vi "Password Protection.vi"(7 "Action (Validate)":T1=enum."Validate Password", 8 "error in":errorcluster, 11 "configuration file path":path) -> (0 "error out":errorcluster, 3 "Validated?":bool)   [LabVIEW 2018, in "Password Protection.lvlib"]
uses:
  Password Protection.lvlib
  Controls/State Machine.ctl
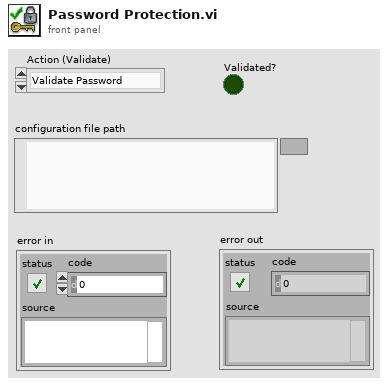
[diagram p1: front panel]
types:
  T1 = typedef "Password Protection.lvlib/State Machine.ctl" = enum16{"Prompt for Password", "Validate Password", "Check Expiration", "Renew Expiration", "Logout", "Stop"}
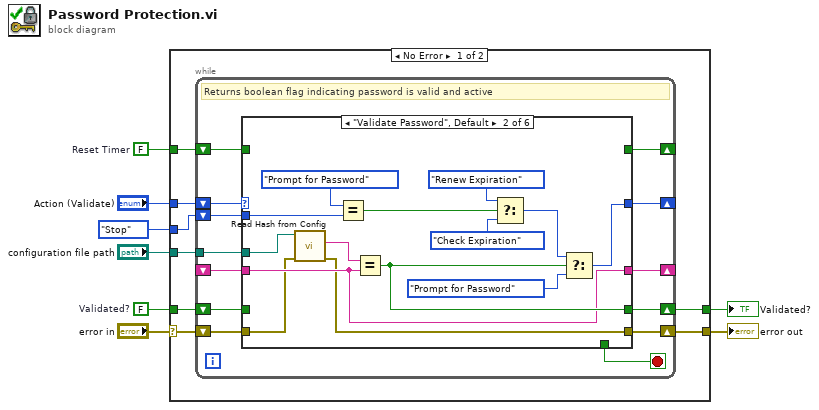
[diagram p0: block diagram]
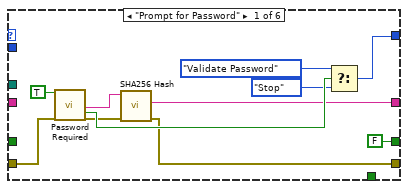
[diagram p2: hidden frame]
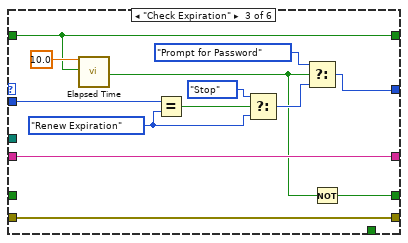
[diagram p3: hidden frame]
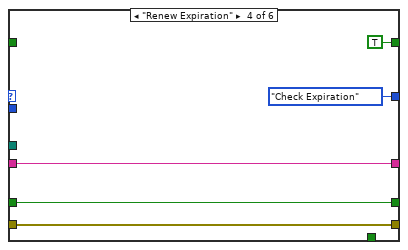
[diagram p4: hidden frame]
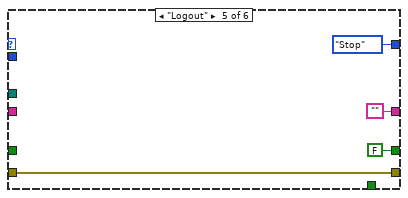
[diagram p5: hidden frame]
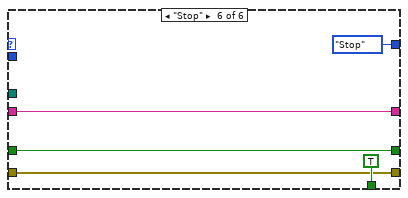
[diagram p6: hidden frame]
diagram:
  w5 = FALSE  # Reset Timer
  w7 = FALSE  # Validated?
  n1 = case shown="No Error" "error in" {
    selector: "error in" -> [w9 w82]
    tunnel: "Action (Validate)" -> [w16 _]
    tunnel: w7 -> [w15 _]
    tunnel: [w14 _] -> w6
    tunnel: w5 -> [w13 _]
    tunnel: State_Machine."Stop" ("f") -> [w12 _]
    tunnel: "configuration file path" -> [w11 _]
    tunnel: [w10 w82] -> w1
    frame No Error {
      n2 = while {
        shift-right: [w28] -> _
        shift-left: _ -> [w29]
        shift-right: [w26] -> _
        shift-left: w16 -> [w27]
        shift-right: [w24] -> w14
        shift-left: w15 -> [w25]
        shift-right: [w22] -> _
        shift-left: w13 -> [w23]
        shift-left: w12 -> [w21]
        tunnel: w11 -> [w19]
        shift-right: [w18] -> w10
        shift-left: w9 -> [w17]
        stop <- w20 stop-if-true
        # "Returns boolean flag indicating password is valid and active"
        n3 = case shown="\"Validate Password\", Default" w27 {
          tunnel: w29 -> [_ w45 w59 w70 _ w80]
          tunnel: [w33 w45 w59 w70 "" ("Password") w80] -> w28
          tunnel: [w37 w53 w56 State_Machine."Check Expiration" ("f") State_Machine."Stop" ("f") State_Machine."Stop" ("f")] -> w26
          tunnel: w25 -> [_ _ _ w71 _ w81]
          tunnel: [FALSE w52 w57 w71 FALSE ("Validated?") w81] -> w24
          tunnel: w23 -> [_ _ w66 _ _ _]
          tunnel: [_ _ w66 TRUE ("Reset Timer") _ _] -> w22
          tunnel: w21 -> [_ w51 w64 _ _ _]
          tunnel: [_ _ _ _ _ TRUE] -> w20
          tunnel: w19 -> [_ w43 _ _ _ _]
          tunnel: [w31 w41 w55 w68 w73 w77] -> w18
          tunnel: w17 -> [w30 w42 w55 w68 w73 w77]
          frame "Prompt for Password" {
            n4 = call "Password Required"("Enable"=TRUE, "error in (no error)"=w30) -> ("Password"=w34:string, "OK"=w39:bool, "error out"=w32:errorcluster)  [unwired: 15 in]
            n5 = call "SHA256 Hash.vi"("error in"=w32, "String"=w34) -> ("error out"=w31:errorcluster, "hash"=w33:string)  [unwired: 8 in]
            n6 = Select(t=State_Machine."Validate Password", s=w39, f=State_Machine."Stop") -> (s? t:f=w37:T1)
          }
          frame "Validate Password", Default {
            n7 = call "Read Hash from Config.vi"("error in"=w42, "configuration file path"=w43) -> ("error out"=w41:errorcluster, "hash"=w44:string)  [unwired: 8 in]
            n8 = Equal?(x=State_Machine."Prompt for Password", y=w51) -> (x = y?=w49:bool)
            n9 = Equal?(x=w44, y=w45) -> (x = y?=w52:bool)
            n10 = Select(t=State_Machine."Renew Expiration", s=w49, f=State_Machine."Check Expiration" ("t")) -> (s? t:f=w46:T1)
            n11 = Select(t=w46, s=w52, f=State_Machine."Prompt for Password") -> (s? t:f=w53:T1)
          }
          frame "Check Expiration" {
            w62 = State_Machine."Renew Expiration" ("f")
            n12 = call "Elapsed Time"("Time Target (s)"=10.0, "Reset"=w66) -> ("Time has Elapsed"=w58:bool)  [unwired: 10 in, 7 out]
            n13 = Equal?(x=w64, y=w62) -> (x = y?=w63:bool)
            n14 = Select(t=State_Machine."Stop", s=w63, f=w62) -> (s? t:f=w61:T1)
            n15 = Select(t=State_Machine."Prompt for Password" ("f"), s=w58, f=w61) -> (s? t:f=w56:T1)
            n16 = Not(x=w58) -> (.not. x?=w57:bool)
          }
          frame "Renew Expiration" {
          }
          frame "Logout" {
          }
          frame "Stop" {
          }
        }
      }
    }
    frame Error {
    }
  }
  "Validated?" <- w6
  "error out" <- w1
